vi "GUI_SRS_PS300.vi"() -> ()   [LabVIEW 2013]
uses:
  Shared/GUI_Template/GUI_master/tcp_new_data_event.ctl
  Shared/GUI_Template/GUI_master/tcp new data cluster.ctl
panel:
  in  "GUIdevice 2":string="TPS_HVPHOS"
  in  "stop":bool
  out "volts 2":dbl(graph) caption="Waveform Chart 2"
  in  "Voltage set 2":dbl caption="Voltage set" min=-1000.0 max=0.0 format="%_4p"
  in  "High Voltage::2":bool caption="High Voltage On/Off"
  in  "Reset::2":bool caption="Reset"
  out "ampere 2":dbl(graph)
  in  "Current::2":dbl=29.9701 caption="Current (A)" min=0.0 max=0.2 format="%_4p"
  in  "Voltage::2":dbl=29.9701 caption="Voltage (V)" min=0.0 max=4000.0 format="%_4p"
  in  "Trip Current::2":dbl=29.9701 caption="Trip Current (A)" min=0.0 max=0.01 format="%_4p"
  out "volts":dbl(graph) caption="Waveform Chart 2"
  in  "Voltage set":dbl min=-1000.0 max=0.0 format="%_4p"
  in  "High Voltage::1":bool caption="High Voltage On/Off"
  in  "Reset::1":bool caption="Reset"
  out "ampere":dbl(graph)
  in  "Current::1":dbl=29.9701 caption="Current (A)" min=0.0 max=0.2 format="%_4p"
  in  "Voltage::1":dbl=29.9701 caption="Voltage (V)" min=-1000.0 max=0.0 format="%_4p"
  in  "Trip Current::1":dbl=29.9701 caption="Trip Current (A)" min=0.0 max=0.01 format="%_4p"
  in  "GUIdevice 1":string="TPS_HVMCP"
  in  "insert tag":bool=TRUE
  out "tcp data event":T1
  out "error IO 2":errorcluster
  # "MCP High Voltage Control (-1000V to 0)"
  # "Phosphor High Voltage Control (0 to 4000V)"
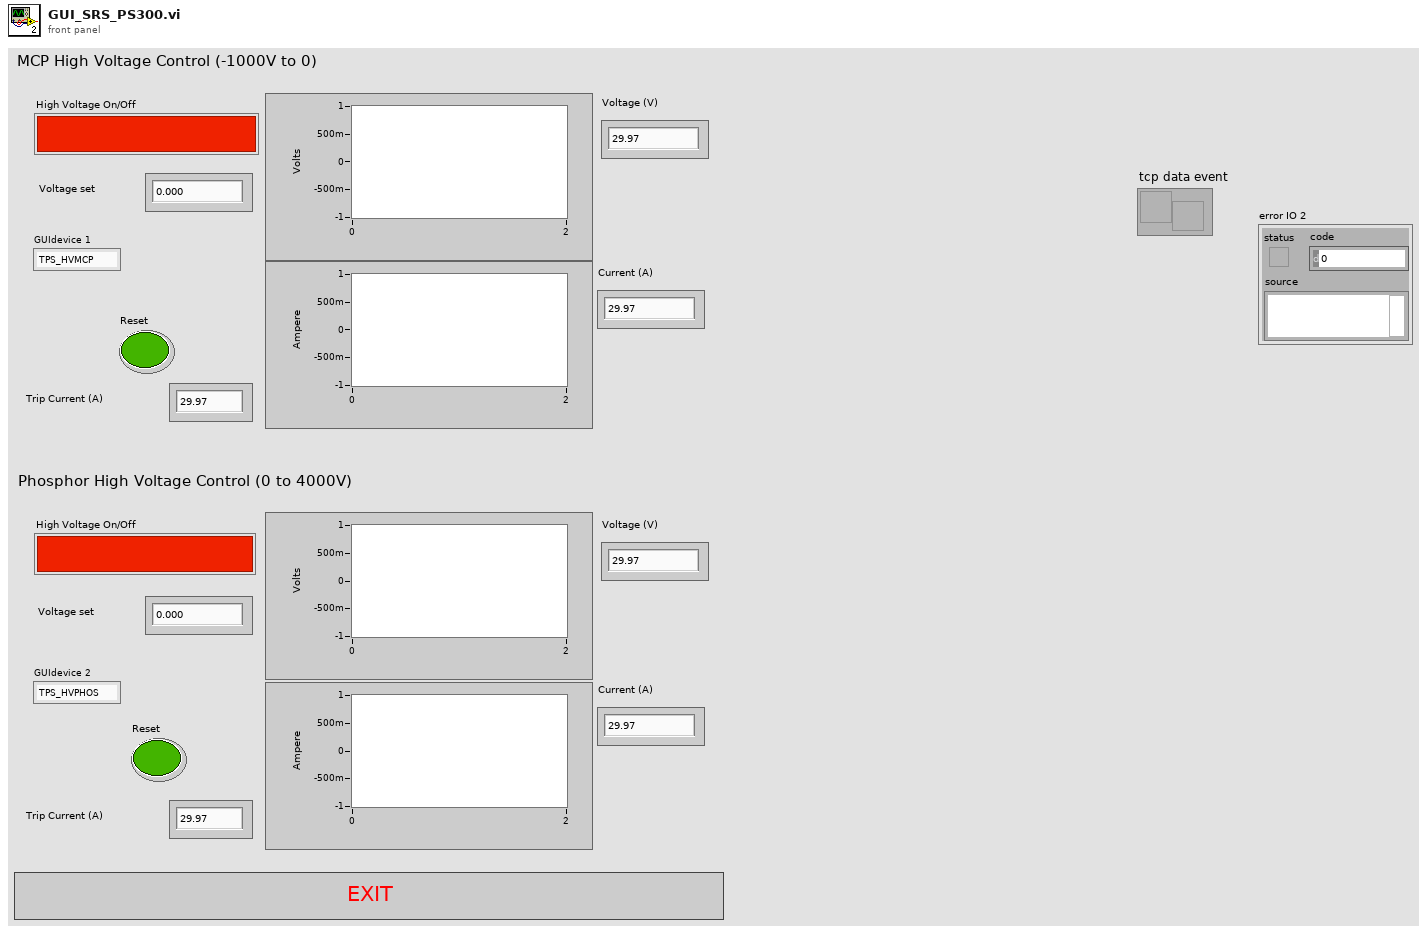
[diagram p1: front panel]
types:
  T1 = typedef "tcp_new_data_event.ctl" = refnum<user-event>
  T2 = typedef "tcp new data cluster.ctl" = cluster{"EventEnum":enum16{"new data", "connection status update"}, "Device name":string}
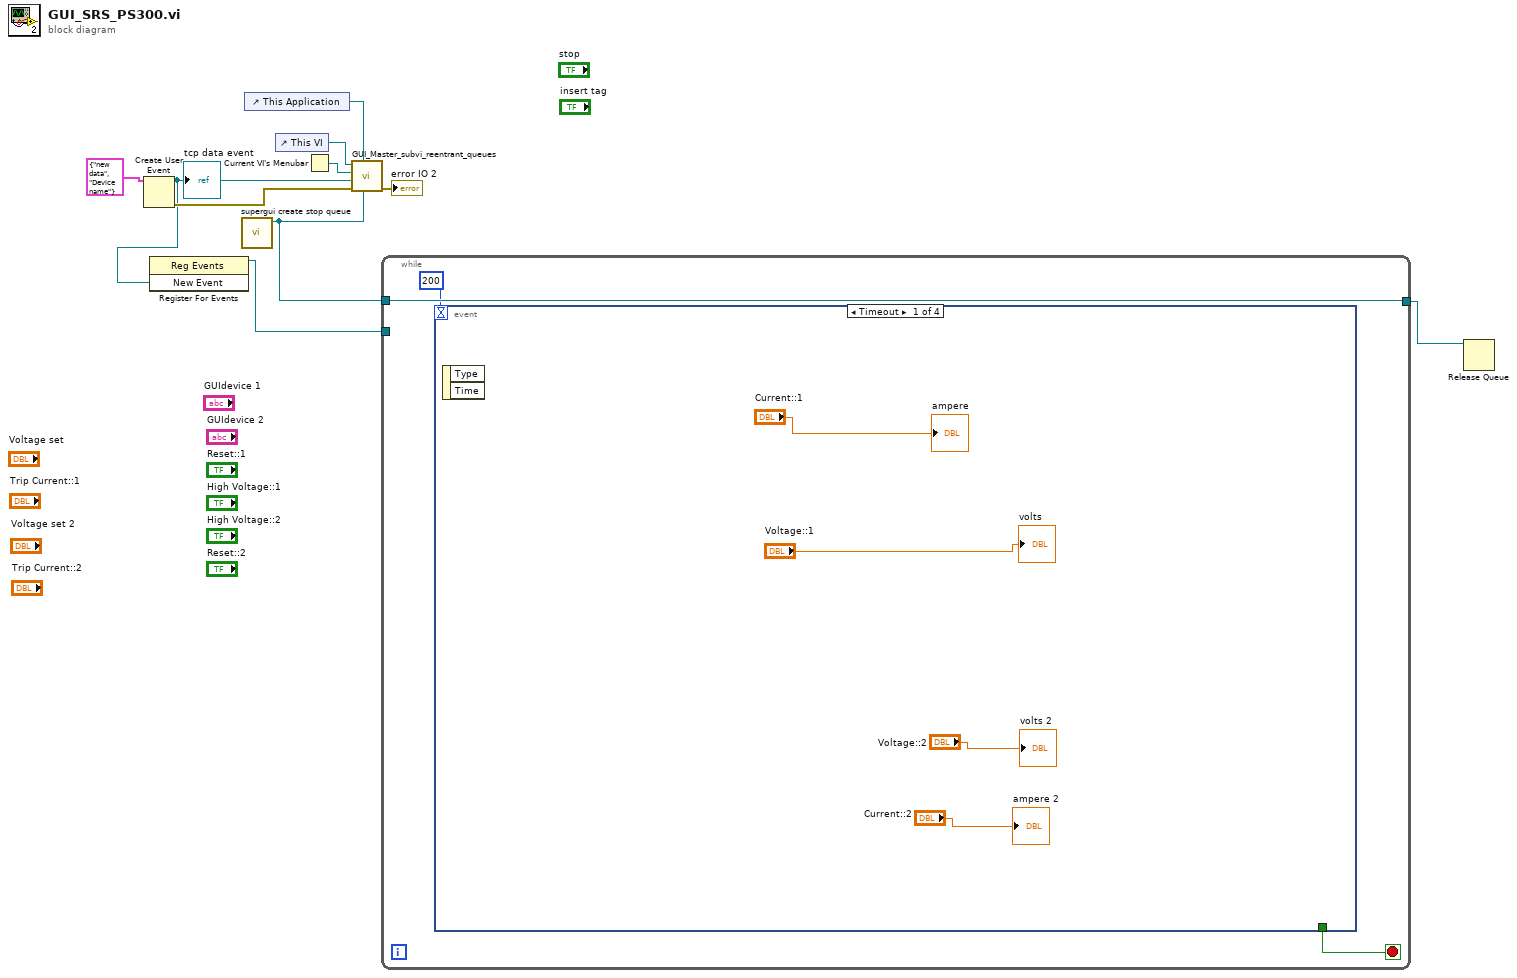
[diagram p0: block diagram]
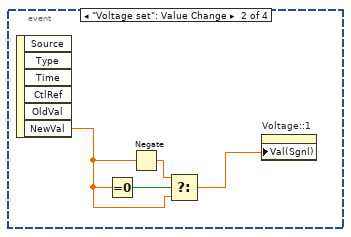
[diagram p2: hidden frame]
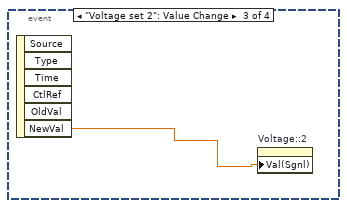
[diagram p3: hidden frame]
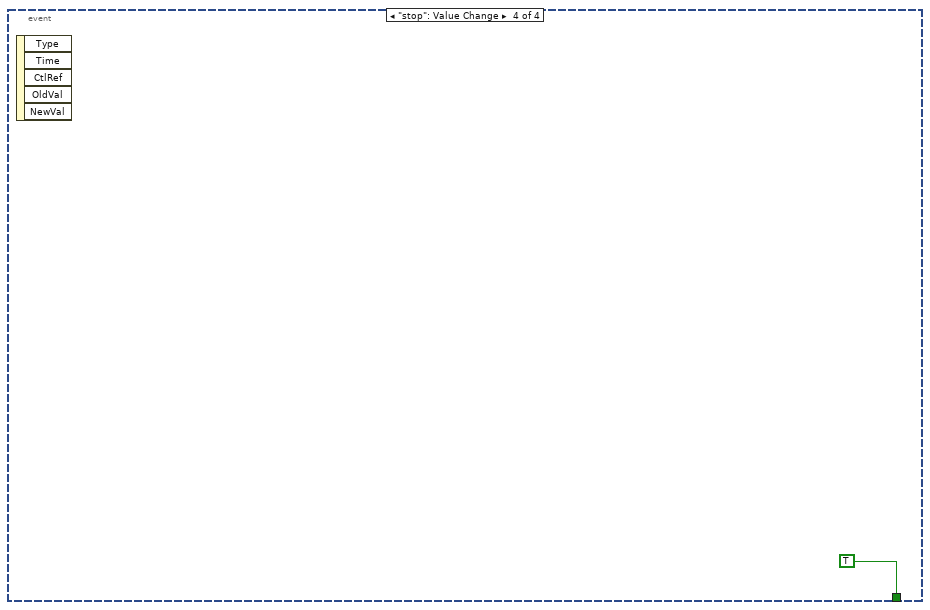
[diagram p4: hidden frame]
diagram:
  n1 = Create User Event(user event datatype=T2 {"EventEnum"=enum."new data", "Device name"="Device name"} ("New Event")) -> (user event=w4:refnum<user-event>, error out=w6:errorcluster)  [unwired: 1 in]
  "tcp data event" <- w4
  n2 = register-events(w4) -> (reference out=w3:refnum<event-registration>)  [unwired: 2 in, 1 out]
  n3 = call "supergui create stop queue.vi"() -> ("STOP Queue out"=w2:refnum<queue>)  [unwired: 11 in]
  n4 = control-ref of="This Application"() -> (w5:refnum<vi>)
  n5 = control-ref of="This VI"() -> (w9:refnum<vi>)
  n6 = Current VI's Menubar() -> (w8:refnum<k9>)
  n7 = call "GUI_Master_subvi_reentrant_queues.vi"("STOP Queue in"=w2, "This Application"=w5, "error in (no error)"=w6, "tcp data event"=w4, "Caller menu reference"=w8, "Caller VI ref"=w9) -> ("error out"=→"error IO 2":errorcluster)  [unwired: 5 in]
  n8 = while {
    tunnel: w3 -> [_]
    tunnel: w2 -> [w12]
    tunnel: [w12] -> w1
    stop <- w13 stop-if-true
    n9 = event shown="[0] Timeout" {
      selector: _ -> [_ _ _ _]
      dyn-events: _ -> [_ _ _ _]
      timeout: 200 ("wait") -> [_ _ _ _]
      tunnel: [_ _ _ TRUE] -> w13
      event Timeout {
        n10 = event-data() -> ()  [unwired: 1 in, 2 out]
        "ampere" <- "Current::1"
        "volts" <- "Voltage::1"
        "volts 2" <- "Voltage::2"
        "ampere 2" <- "Current::2"
      }
      event "Voltage set": Value Change {
        n11 = event-data() -> ("NewVal"=w19:dbl)  [unwired: 1 in, 5 out]
        n12 = Equal To 0?(x=w19) -> (x = 0?=w21:bool)
        n13 = Negate(x=w19) -> (-x=w20:dbl)
        n14 = Select(t=w20, s=w21, f=w19) -> (s? t:f=w18:dbl)
        n15 = property on="Voltage::1" class="DigNum (strict)"("Val(Sgnl)"=w18) -> ()  [unwired: 2 in, 2 out]
      }
      event "Voltage set 2": Value Change {
        n16 = event-data() -> ("NewVal"=w22:dbl)  [unwired: 1 in, 5 out]
        n17 = property on="Voltage::2" class="DigNum (strict)"("Val(Sgnl)"=w22) -> ()  [unwired: 2 in, 2 out]
      }
      event "stop": Value Change {
        n18 = event-data() -> ()  [unwired: 1 in, 5 out]
      }
    }
  }
  n19 = Release Queue(queue=w1) -> ()  [unwired: 2 in, 3 out]
